vi "PMX_ActivateTEDs.vi"(8 "Error in":errorcluster, 10 "Connector":refnum<k24>, 11 "Device":refnum<k24>) -> (0 "Error out":errorcluster, 2 "Result":bool, 3 "Device":refnum<k24>)   [LabVIEW 2016]
doc: "Loads and activates TEDs settings at given connector.\nOn success, the sensor object of the given connector will be replaced by an updated version according to TEDs settings\n\nConnector: Connector to which the TEDs is connected\nResult: True, if TEDs settings could be loaded and activated"
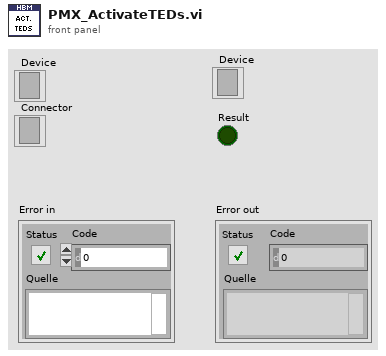
[diagram p1: front panel]
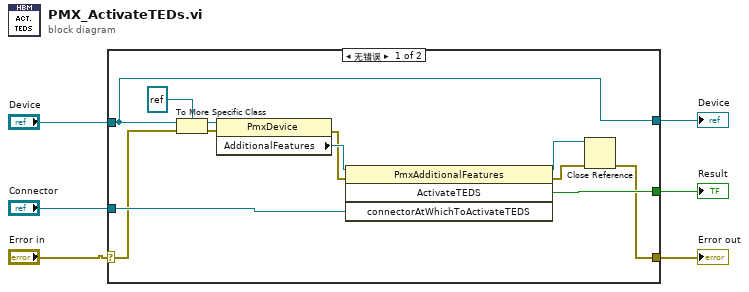
[diagram p0: block diagram]
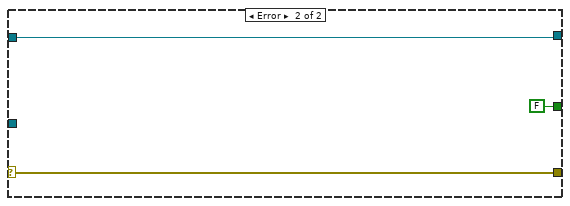
[diagram p2: hidden frame]
diagram:
  n1 = case shown="无错误" "Error in" {
    selector: "Error in" -> [w11 w21]
    tunnel: [w7 w21] -> w3
    tunnel: "Device" -> [w13 w20]
    tunnel: [w14 FALSE ("ActivateTEDS")] -> w2
    tunnel: [w13 w20] -> w4
    tunnel: "Connector" -> [w12 _]
    frame No Error {
      n2 = To More Specific Class(target class=refnum<k24> refnum ("Zielklasse"), reference=w13, error in=w11) -> (specific class reference=w18:refnum<k24>, error out=w15:errorcluster)
      n3 = property on="Eigenschaftsknoten" class="PmxDevice"(reference=w18, error in=w15) -> (error out=w16:errorcluster, "AdditionalFeatures"=w17:refnum<k24>)  [unwired: 1 out]
      n4 = invoke on="Methodenknoten" class="PmxAdditionalFeatures" method="ActivateTEDS"(reference=w17, error in=w16, "connectorAtWhichToActivateTEDS"=w12) -> (reference out=w8:refnum<k24>, error out=w9:errorcluster, "ActivateTEDS"=w14:bool)  [unwired: 1 in, 1 out]
      n5 = Close Reference(reference=w8, error in (no error)=w9) -> (error out=w7:errorcluster)
    }
    frame Error {
    }
  }
  "Device" <- w4
  "Error out" <- w3
  "Result" <- w2
